vi "StartVI.vi"(0 "Label":string, 11 "error in":errorcluster) -> (6 "Application Ref out":refnum<vi>, 8 "VI Reference":refnum<vi>, 15 "error out":errorcluster)   [LabVIEW 2016]
uses:
  Car Wash 16.0/Car Wash.vi
  main/apis/Setup/GetVI/GetVIByPath.vi
  <vilib>/addons/_JKI Toolkits/Caraya/classes/Test/Test.lvclass
  Car Wash 16.0/Car Wash.lvlib
  main/apis/Setup/GetVI/GetVI.lvlib
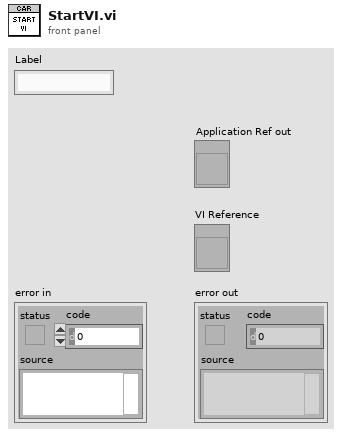
[diagram p1: front panel]
types:
  T1 = enum32{"Invalid", "Standard", "Closed", "Hidden", "Minimized", "Maximized"}
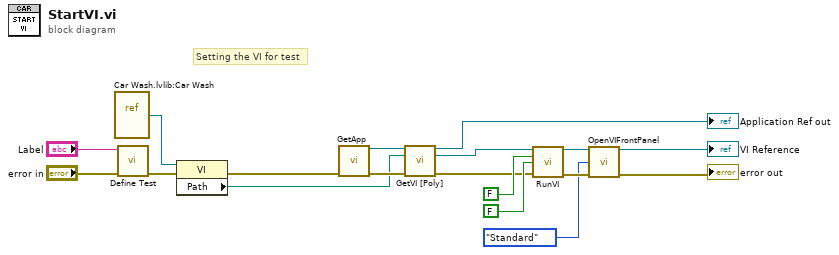
[diagram p0: block diagram]
diagram:
  # "Setting the VI for test"
  n1 = vi-ref "Car Wash.lvlib:Car Wash.vi"() -> (w1:refnum<vi>)
  n2 = call <vilib>:"Define Test.vi"("error in (no error)"="error in", "Label (VI Title)"="Label") -> ("error out"=w2:errorcluster)  [unwired: 9 in]
  n3 = property on="Property Node" class="VI"(reference=w1, error in=w2) -> (error out=w18:errorcluster, "Path"=w15:path)  [unwired: 1 out]
  n4 = call "GetApp.vi"("error in (no error)"=w18) -> ("Application Ref"=w16:refnum<vi>, "error out"=w17:errorcluster)  [unwired: 13 in]
  n5 = call-poly "GetVI [Poly].vi"("Application Ref in"=w16, "VI Path"=w15, "error in (no error)"=w17) -> ("Application Ref out"=→"Application Ref out":refnum<vi>, "VI Reference"=w3:refnum<vi>, "error out"=w6:errorcluster)  [unwired: 10 in]
  n6 = call "RunVI.vi"("VI Reference In"=w3, "Wait Until Done (F)"=FALSE ("Wait Until Done"), "Auto Dispose Reference (F)"=FALSE ("Auto Dispose Reference"), "error in"=w6) -> ("VI Reference Out"=w8:refnum<vi>, "error out"=w9:errorcluster)  [unwired: 10 in]
  n7 = call "OpenVIFrontPanel.vi"("VI Reference In"=w8, "State(Standard)"=T1."Standard" ("State"), "error in"=w9) -> ("VI Reference Out"=→"VI Reference":refnum<vi>, "error out"=→"error out":errorcluster)  [unwired: 11 in]
